vi "scale.vi"(9 "Scale":string, 10 "Center":string, 11 "data":dbl[][](array[numeric])) -> (3 "data (scaled)":dbl[][](array[numeric]))   [LabVIEW 2014]
uses:
  <vilib>/Analysis/baseanly.llb/Mean (DBL).vi
  <vilib>/Analysis/5stat.llb/RMS (DBL).vi
  <vilib>/Analysis/NI_AALBase.lvlib
  <vilib>/Analysis/NI_AALPro.lvlib
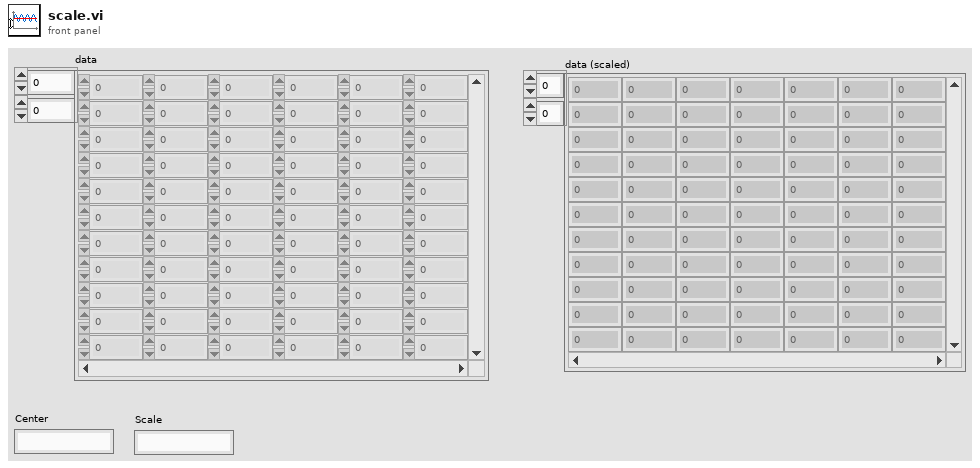
[diagram p1: front panel]
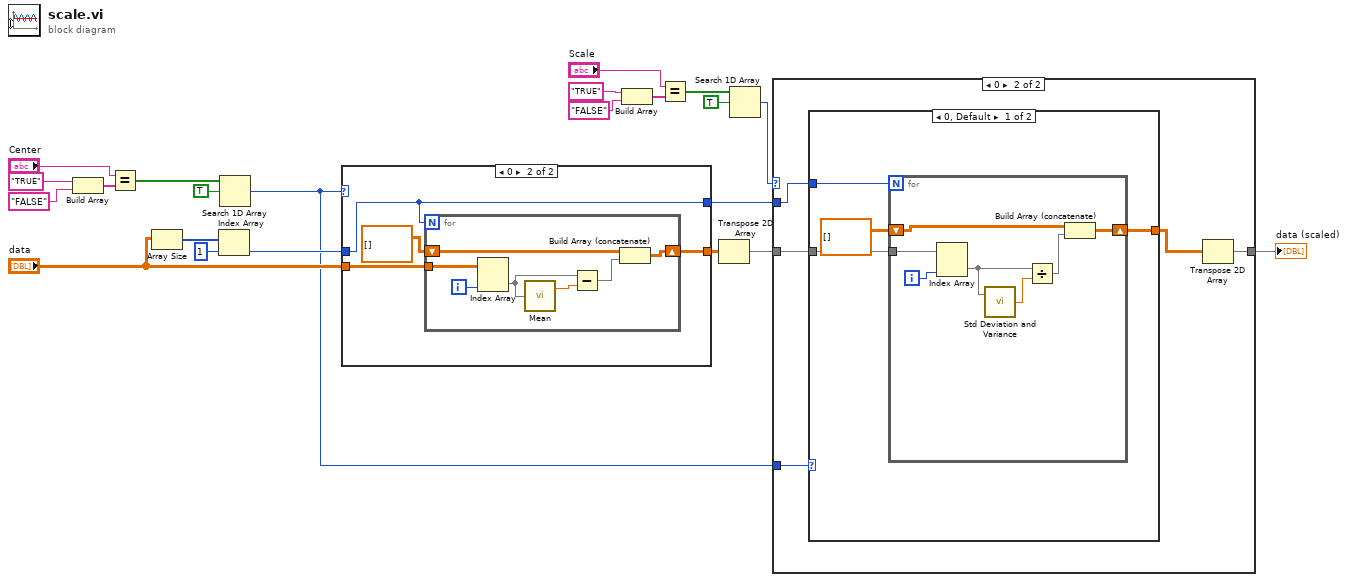
[diagram p0: block diagram]
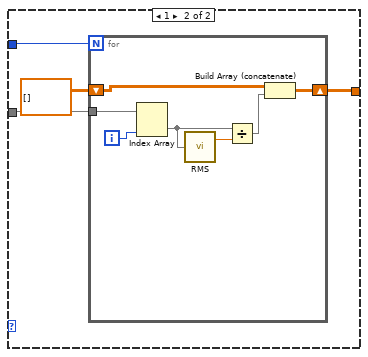
[diagram p3: hidden frame]
diagram:
  n1 = Build Array("TRUE" ("y"), "FALSE") -> (w17:string[])
  n2 = Equal?(x="Center", y=w17) -> (x = y?=w15:bool[])
  n3 = Array Size(array="data") -> (size(s)=w22:i32[])
  n4 = Index Array(array=w22, index=1) -> (element=w20:i32)
  n5 = Search 1D Array(1D array=w15, element=TRUE) -> (index of element=w3:i32)  [unwired: 1 in]
  n6 = case shown="0" w3 {
    tunnel: w20 -> [w23 w25]
    tunnel: "data" -> [w24 w27]
    tunnel: [w24 w26] -> w6
    tunnel: [w23 w25] -> w5
    frame 1, Default {
    }
    frame 0 {
      n7 = for {
        N: w25 -> [_]
        tunnel: w27 -> [w35]
        shift-right: [w32] -> w26
        shift-left: dbl[][] [] -> [w31]
        i -> [w34]
        n8 = Index Array(array=w35, index (col)=w34) -> (element=w29:dbl[])  [unwired: 1 in]
        n9 = call-poly <vilib>:"Mean.vi"("X"=w29) -> ("mean"=w30:dbl)  [unwired: 1 out]
        n10 = Subtract(x=w29, y=w30) -> (x-y=w33:dbl[])
        n11 = Build Array (concatenate)(w31, w33) -> (w32:dbl[][])
      }
    }
  }
  n12 = Build Array("TRUE" ("y"), "FALSE") -> (w12:string[])
  n13 = Equal?(x="Scale", y=w12) -> (x = y?=w7:bool[])
  n14 = Transpose 2D Array(2D array=w6) -> (transposed array=w1:dbl[][])
  n15 = Search 1D Array(1D array=w7, element=TRUE) -> (index of element=w4:i32)  [unwired: 1 in]
  n16 = case shown="0" w4 {
    tunnel: w5 -> [_ w37]
    tunnel: w1 -> [w36 w40]
    tunnel: [w36 w38] -> w2
    tunnel: w3 -> [_ w41]
    frame 1, Default {
    }
    frame 0 {
      n17 = case shown="0, Default" w41 {
        tunnel: w40 -> [w44 w55]
        tunnel: w37 -> [w45 w54]
        tunnel: [w42 w53] -> w39
        frame 0, Default {
          n18 = for {
            N: w45 -> [_]
            tunnel: w44 -> [w52]
            shift-right: [w48] -> w42
            shift-left: dbl[][] [] -> [w47]
            i -> [w51]
            n19 = Index Array(array=w52, index (col)=w51) -> (element=w50:dbl[])  [unwired: 1 in]
            n20 = call <vilib>:"Std Deviation and Variance.vi"("X"=w50) -> ("standard deviation"=w46:dbl)  [unwired: 1 in, 2 out]
            n21 = Divide(x=w50, y=w46) -> (x/y=w49:dbl[])
            n22 = Build Array (concatenate)(w47, w49) -> (w48:dbl[][])
          }
        }
        frame 1 {
          n23 = for {
            N: w54 -> [_]
            tunnel: w55 -> [w63]
            shift-right: [w60] -> w53
            shift-left: dbl[][] [] -> [w59]
            i -> [w62]
            n24 = Index Array(array=w63, index (col)=w62) -> (element=w57:dbl[])  [unwired: 1 in]
            n25 = call-poly <vilib>:"RMS.vi"("X"=w57) -> ("rms value"=w58:dbl)  [unwired: 1 out]
            n26 = Divide(x=w57, y=w58) -> (x/y=w61:dbl[])
            n27 = Build Array (concatenate)(w59, w61) -> (w60:dbl[][])
          }
        }
      }
      n28 = Transpose 2D Array(2D array=w39) -> (transposed array=w38:dbl[][])
    }
  }
  "data (scaled)" <- w2
